vi "_ DB Delete Tables.vi"() -> ()   [LabVIEW 2012]
uses:
  DB Connection Mode enum.ctl
  Database Lib.lvlib
  Utility/database/NI_Database_API_64.lvlib
panel:
  out "error out":errorcluster
  out "tables":string[](array[string])
  # "When Run, Each Found Table will be prompted to be deleted from the database"
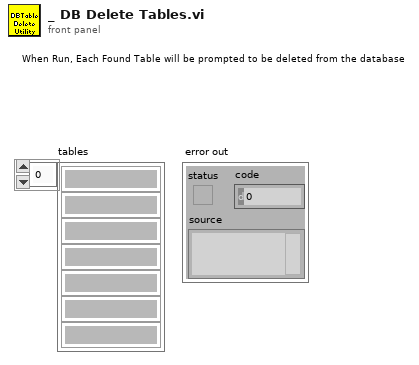
[diagram p1: front panel]
types:
  T1 = typedef "Database Lib.lvlib/DB Connection Mode enum.ctl" = enum16{"Connect", "Get Connection", "Disconnect"}
  T2 = typedef "NI_Database_API_64.lvlib/Conn ObjectReference.ctl" = refnum<k1>
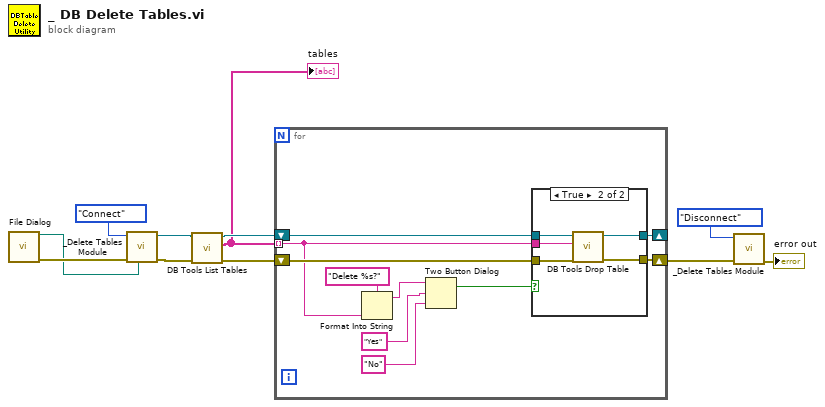
[diagram p0: block diagram]
diagram:
  n1 = call "File Dialog"() -> ("selected path"=w1:path, "error out"=w3:errorcluster)  [unwired: 7 in, 7 out]
  n2 = call "_Delete Tables Module.vi"("connection information"=w1, "error in (no error)"=w3, "Mode (Get Connection)"=DB_Connection_Mode_enum."Connect" ("Mode")) -> ("error out"=w4:errorcluster, "connection reference"=w5:T2)  [unwired: 7 out]
  n3 = call "DB Tools List Tables.vi"("error in (no error)"=w4, "connection reference"=w5) -> ("error out"=w9:errorcluster, "tables"=w7:string[], "connection reference out"=w10:T2)  [unwired: 3 out]
  "tables" <- w7
  n4 = for {
    shift-right: [w19] -> _
    shift-left: w10 -> [w21]
    shift-right: [w18] -> w8
    shift-left: w9 -> [w20]
    tunnel: w7 -> [w15] mode=indexing
    n5 = Format Into String(format string="Delete %s?", w15) -> (resulting string=w14:string)  [unwired: 2 in, 1 out]
    n6 = Two Button Dialog(message=w14, 1:"No" ("F button name (\"Cancel\")"), 2:"Yes" ("F button name (\"Cancel\")")) -> (T button?=w17:bool)
    n7 = case shown="True" w17 {
      tunnel: w21 -> [w23 w28]
      tunnel: w20 -> [w22 w27]
      tunnel: [w23 w26] -> w19
      tunnel: [w22 w25] -> w18
      tunnel: w15 -> [_ w24]
      frame False {
      }
      frame True {
        n8 = call "DB Tools Drop Table.vi"("error in (no error)"=w27, "table"=w24, "connection reference"=w28) -> ("error out"=w25:errorcluster, "connection reference out"=w26:T2)  [unwired: 5 out]
      }
    }
  }
  n9 = call "_Delete Tables Module.vi"("error in (no error)"=w8, "Mode (Get Connection)"=DB_Connection_Mode_enum."Disconnect" ("Mode")) -> ("error out"=→"error out":errorcluster)  [unwired: 1 in, 8 out]
